vi "003LockerComboAns.vi"() -> ()   [LabVIEW 2010]
panel:
  out "Can Open?":bool
  in  "#4":i32
  in  "#3":i32
  in  "#2":i32
  in  "#1":i32
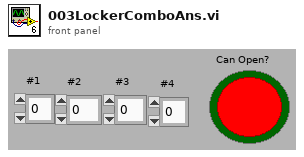
[diagram p1: front panel]
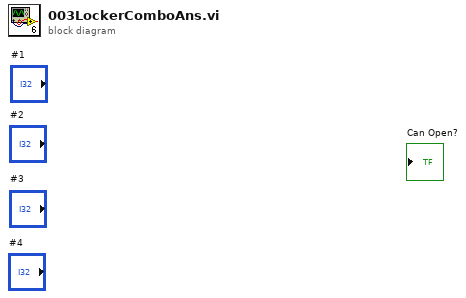
[diagram p0: block diagram]
diagram:
